vi "ClsConfigureInitValues.vi"(8 "error in (no error)":errorcluster, 10 "InitCommandArray":string[](array[string]), 11 "Connection Out in in":u32) -> (0 "error out":errorcluster, 2 "Out":T1, 3 "Connection Out out 2":u32)   [LabVIEW 2015]
uses:
  TypeDefs/ClsConfigureValues.ctl
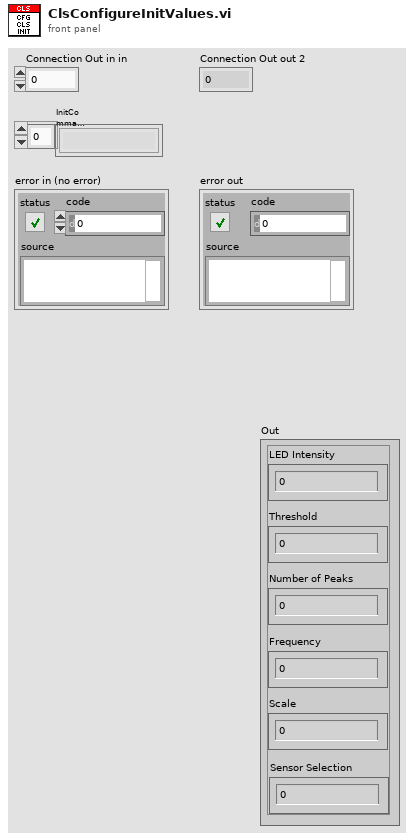
[diagram p1: front panel]
types:
  T1 = typedef "ClsConfigureValues.ctl" = cluster{"LED Intensity":i32, "Threshold":i32, "Number of Peaks":i32, "Frequency":i32, "Scale":i32, "Sensor Selection":i32}
  T2 = cluster{"[0]":i32, "[1]":i32, "[2]":i32, "[3]":i32, "[4]":i32}
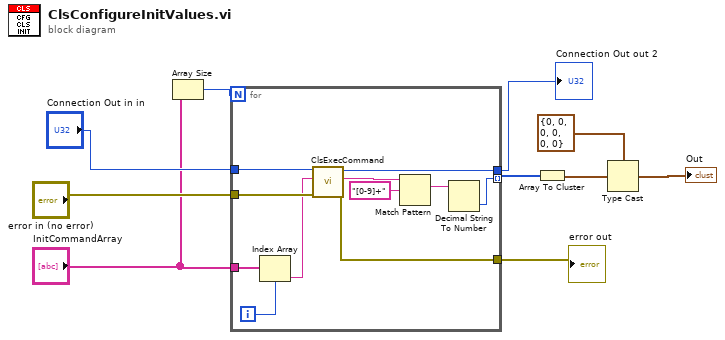
[diagram p0: block diagram]
diagram:
  n1 = Array Size(array="InitCommandArray") -> (size(s)=w6:i32)
  n2 = for {
    N: w6 -> [_]
    tunnel: "error in (no error)" -> [w21]
    tunnel: [w14] -> w9
    tunnel: [w20] -> w8
    tunnel: "Connection Out in in" -> [w19]
    tunnel: "InitCommandArray" -> [w17]
    tunnel: [w11] -> w4 mode=indexing
    i -> [w18]
    n3 = Index Array(array=w17, index=w18) -> (element=w16:string)
    n4 = call "ClsExecCommand.vi"("error in (no error)"=w21, "Command In"=w16, "Connection In"=w19) -> ("error out"=w14:errorcluster, "Command Response"=w15:string, "Connection Out"=w20:u32)  [unwired: 6 in]
    n5 = Match Pattern(string=w15, regular expression="[0-9]+") -> (match substring=w12:string)  [unwired: 1 in, 3 out]
    n6 = Decimal String To Number(string=w12) -> (number=w11:i32)  [unwired: 2 in, 1 out]
  }
  "Connection Out out 2" <- w8
  "error out" <- w9
  n7 = Array To Cluster(array=w4) -> (cluster=w3:T2)
  n8 = Type Cast(type=T1 {"LED Intensity"=0, "Threshold"=0, "Number of Peaks"=0, "Frequency"=0, "Scale"=0, "Sensor Selection"=0} ("ClsConfigureValues"), x=w3) -> (*(type *) &x=→"Out":T1)
